vi "get channels test.vi"() -> (0 "error out":errorcluster, 3 "channels match":bool)   [LabVIEW 2018, in "Add Module tests.lvlib"]
doc: "Tests the 'Get Channels' VI of the Configuration class."
uses:
  Add Module tests.lvlib
  module/configuration/Add Module configuration.lvclass
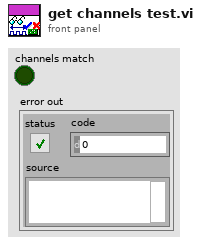
[diagram p1: front panel]
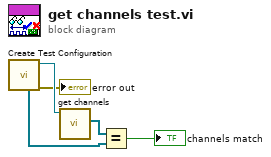
[diagram p0: block diagram]
diagram:
  n1 = call "Create Test Configuration.vi"() -> ("error out"=→"error out":errorcluster, "Module Configuration"=w5:refnum<class "Add Module configuration.lvclass">, "Channels"=w2:refnum<class "TBM channel.lvclass">[])  [unwired: 6 in, 3 out]
  n2 = call-dynamic "get channels.vi"("Add Module configuration in"=w5) -> ("channels"=w3:refnum<class "TBM channel.lvclass">[])  [unwired: 9 in, 1 out]
  n3 = Equal?(x=w3, y=w2) -> (x = y?=→"channels match":bool)
